vi "TopicRequest_Request.vi"(1 "ROS":T1={"topic port"=0, "Node"="", "topic"="", "type"="", "node port"=0, "error "={"status"=FALSE, "code"=0, "source"=""}, "Direction"=enum."Node", "Update (ms)"=1, "FIFO size"=1}) -> (0 "XML":string)   [LabVIEW 2018]
doc: "Returns the XML required to request a topic"
uses:
  <userlib>/ROS for LabVIEW Software/ROS/Code/SubVIs/_ROSControl.ctl
  <userlib>/ROS for LabVIEW Software/ROS/Code/SubVIs/_ROSDirection.ctl
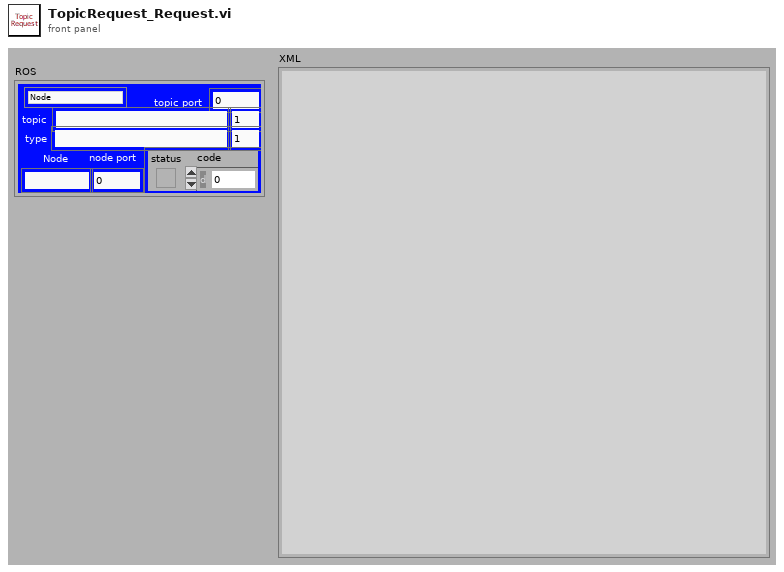
[diagram p1: front panel]
types:
  T1 = typedef "_ROSControl.ctl" = cluster{"topic port":u16, "Node":string, "topic":string, "type":string, "node port":u16, "error ":errorcluster, "Direction":T2, "Update (ms)":u16, "FIFO size":u16}
  T2 = typedef "_ROSDirection.ctl" = enum16{"Node", "Publisher", "Subscriber", "ServiceClient", "ServiceProvider"}
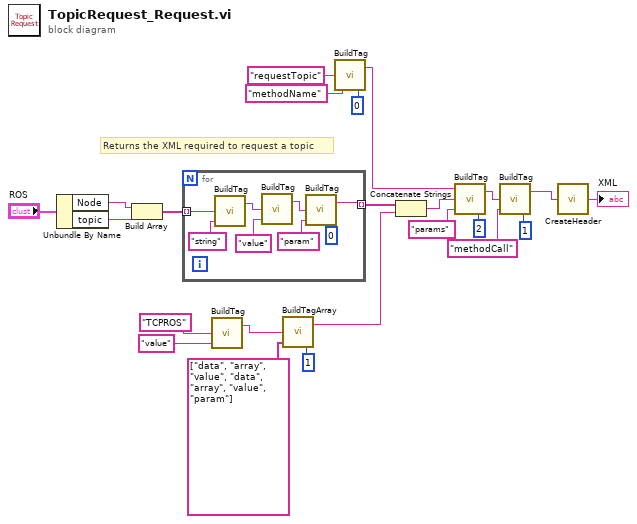
[diagram p0: block diagram]
diagram:
  # "Returns the XML required to request a topic"
  n1 = Unbundle By Name("ROS") -> ("Node"=w22:string, "topic"=w21:string)
  n2 = Build Array(w22, w21) -> (w20:string[])
  n3 = for {
    tunnel: w20 -> [w31] mode=indexing
    tunnel: [w30] -> w19 mode=indexing
    n4 = call <userlib>:"BuildTag.vi"("tag"="string", "value"=w31) -> ("string out"=w28:string)  [unwired: 2 in]
    n5 = call <userlib>:"BuildTag.vi"("tag"="value", "value"=w28) -> ("string out"=w29:string)  [unwired: 2 in]
    n6 = call <userlib>:"BuildTag.vi"("Indent"=i8 0, "tag"="param", "value"=w29) -> ("string out"=w30:string)  [unwired: 1 in]
  }
  n7 = call <userlib>:"BuildTag.vi"("tag"="value", "value"="TCPROS") -> ("string out"=w2:string)  [unwired: 2 in]
  n8 = call <userlib>:"BuildTagArray.vi"("Indent"=i8 1, "tags"=string[] ["data", "array", "value", "data", "array", "value", "param"], "value"=w2) -> ("string out"=w17:string)  [unwired: 1 in]
  n9 = call <userlib>:"BuildTag.vi"("Indent"=i8 0, "tag"="methodName", "value"="requestTopic") -> ("string out"=w13:string)  [unwired: 1 in]
  n10 = Concatenate Strings(w19, w17) -> (w12:string)
  n11 = call <userlib>:"BuildTag.vi"("Indent"=i8 2, "tag"="params", "value"=w12, "string in"=w13) -> ("string out"=w8:string)
  n12 = call <userlib>:"BuildTag.vi"("Indent"=i8 1, "tag"="methodCall", "value"=w8) -> ("string out"=w6:string)  [unwired: 1 in]
  n13 = call <userlib>:"CreateHeader.vi"("Content"=w6) -> ("XML"=→"XML":string)
